vi "Drive Immediate with Angle Control.vi"(7 "Description":string, 8 "Command Info In":T1, 10 "Right Setpoint":dbl, 11 "Left Setpoint":dbl) -> (0 "Command Info Out":T1)   [LabVIEW 2019]
doc: "This VI notifies the subsystem to the new setpoint."
uses:
  Implementation/Drive Operations.ctl
  Implementation/Drive Setpoints.ctl
  <vilib>/Rock Robotics/WPI/Framework/Completion Status.ctl
  <vilib>/Rock Robotics/WPI/Framework/Completion Notifier.ctl
  <vilib>/Rock Robotics/WPI/Framework/Command Status Info.ctl
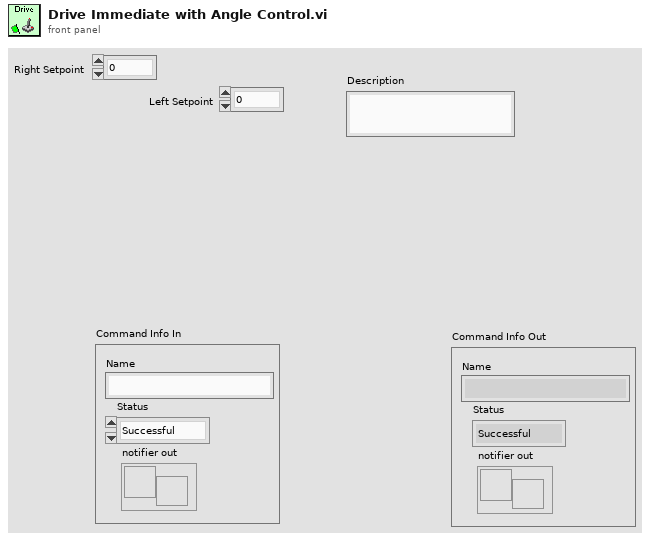
[diagram p1: front panel]
types:
  T1 = typedef "Command Status Info.ctl" = cluster{"Name":string, "Status":T2, "notifier out":T3}
  T2 = typedef "Completion Status.ctl" = enum16{"Successful", "Aborted", "Incomplete"}
  T3 = typedef "Completion Notifier.ctl" = refnum<notifier>
  T4 = typedef "Drive Setpoints.ctl" = cluster{"Operation":T5, "Left Setpoint":dbl, "Right Setpoint":dbl, "Duration":dbl}
  T5 = typedef "Drive Operations.ctl" = enum16{"Reserve", "Drive Immediate with Angle Control", "Read Current", "Immediate", "Drive for Time", "Drive for Distance"}
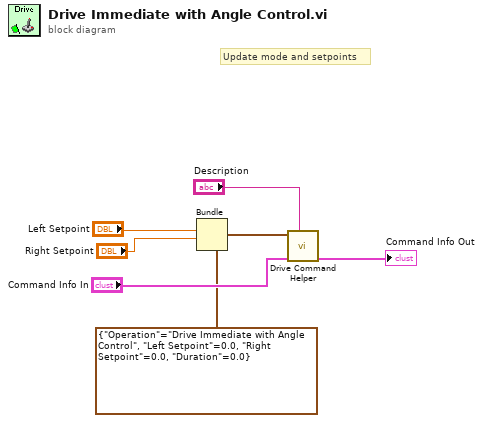
[diagram p0: block diagram]
diagram:
  # "Update mode and setpoints"
  n1 = Bundle(cluster=T4 {"Operation"=enum."Drive Immediate with Angle Control", "Left Setpoint"=0.0, "Right Setpoint"=0.0, "Duration"=0.0} ("SubSystem Data"), "Left Setpoint"="Left Setpoint", "Right Setpoint"="Right Setpoint") -> (w2:T4)  [unwired: 2 in]
  n2 = call "Drive Command Helper.vi"("Description"="Description", "Command Info In"="Command Info In", "SubSystem Data"=w2) -> ("Command Info Out"=→"Command Info Out":T1)  [unwired: 6 in, 2 out]
